vi "Read Measurement.vi"(8 "error in (no error)":errorcluster, 10 "Read From Display (0: Primary)":u16(ring) items=["Primary", "Secondary ", "Both"], 11 "VISA resource name":refnum<visa-resource-name>) -> (0 "error out":errorcluster, 1 "Secondary Display Measurement":dbl, 2 "Primary Display Measurement":dbl, 3 "VISA resource name out":refnum<visa-resource-name>, 4 "Secondary Display Units":string, 5 "Primary Display Units":string)   [LabVIEW 2015, in "Fluke 8808.lvlib"]
doc: "Reads and returns a single measurement from the instrument."
uses:
  <instrlib>/Fluke 8808/Fluke 8808.lvlib
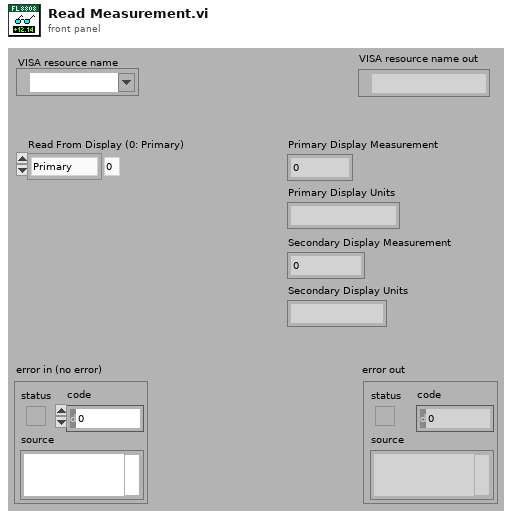
[diagram p1: front panel]
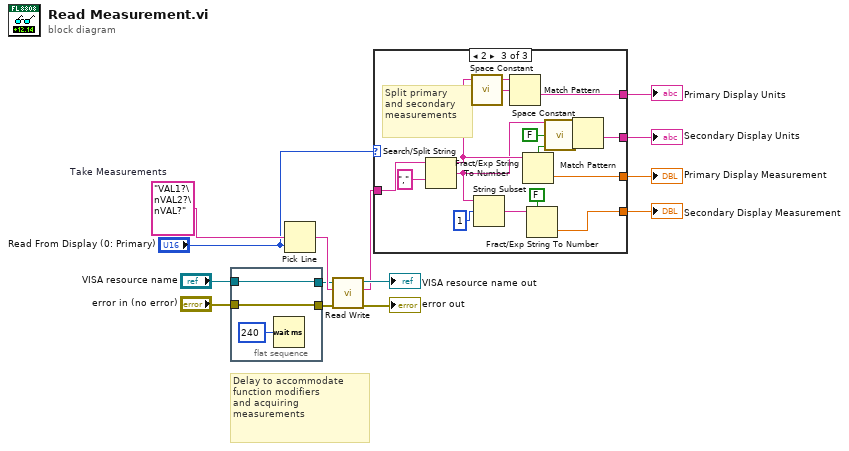
[diagram p0: block diagram]
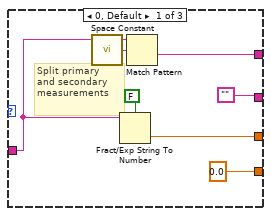
[diagram p2: hidden frame]
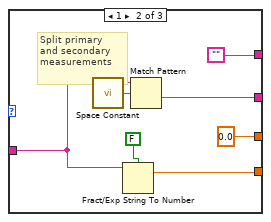
[diagram p3: hidden frame]
diagram:
  w12 = "VAL1?\nVAL2?\nVAL?"  # Take Measurements
  # "Delay to accommodate\nfunction modifiers\nand acquiring\nmeasurements"
  n1 = flat-sequence {
    tunnel: "error in (no error)" -> [w16]
    tunnel: [w16] -> w3
    tunnel: "VISA resource name" -> [w15]
    tunnel: [w15] -> w1
    frame #0 {
      n2 = Wait (ms)(milliseconds to wait=u32 240) -> ()  [unwired: 1 out]
    }
  }
  n3 = Pick Line(multi-line string=w12, line index="Read From Display (0: Primary)") -> (output string=w11:string)  [unwired: 1 in]
  n4 = call <instrlib>:"Read Write.vi"("error in (no error)"=w3, "Write String"=w11, "VISA resource name"=w1) -> ("error out"=→"error out":errorcluster, "Read Data"=w10:string, "VISA resource name out"=→"VISA resource name out":refnum<visa-resource-name>)  [unwired: 6 in]
  n5 = case shown="2" "Read From Display (0: Primary)" {
    tunnel: w10 -> [w21 w29 w45]
    tunnel: [0.0 w26 w35] -> w8
    tunnel: [w19 0.0 w36] -> w7
    tunnel: [w22 "" w41] -> w6
    tunnel: ["" w27 w37] -> w5
    frame 0, Default {
      # "Split primary\nand secondary\nmeasurements"
      n6 = call <vilib>:"Space Constant.vi"() -> ("String"=w20:string)
      n7 = Fract/Exp String To Number(use system decimal point (T)=FALSE, string=w21) -> (number=w19:dbl)  [unwired: 2 in, 1 out]
      n8 = Match Pattern(string=w21, regular expression=w20) -> (after substring=w22:string)  [unwired: 1 in, 3 out]
    }
    frame 1 {
      # "Split primary\nand secondary\nmeasurements"
      n9 = call <vilib>:"Space Constant.vi"() -> ("String"=w30:string)
      n10 = Fract/Exp String To Number(use system decimal point (T)=FALSE, string=w29) -> (number=w26:dbl)  [unwired: 2 in, 1 out]
      n11 = Match Pattern(string=w29, regular expression=w30) -> (after substring=w27:string)  [unwired: 1 in, 3 out]
    }
    frame 2 {
      # "Split primary\nand secondary\nmeasurements"
      n12 = Search/Split String(string=w45, search string/char (-)=",") -> (substring before match=w40:string, match + rest of string=w38:string)  [unwired: 1 in, 1 out]
      n13 = call <vilib>:"Space Constant.vi"() -> ("String"=w39:string)
      n14 = String Subset(string=w38, offset (0)=1) -> (substring=w42:string)  [unwired: 1 in]
      n15 = Match Pattern(string=w40, regular expression=w39) -> (after substring=w41:string)  [unwired: 1 in, 3 out]
      n16 = Fract/Exp String To Number(use system decimal point (T)=FALSE, string=w40) -> (number=w36:dbl)  [unwired: 2 in, 1 out]
      n17 = Fract/Exp String To Number(use system decimal point (T)=FALSE, string=w42) -> (number=w35:dbl)  [unwired: 2 in, 1 out]
      n18 = call <vilib>:"Space Constant.vi"() -> ("String"=w34:string)
      n19 = Match Pattern(string=w38, regular expression=w34) -> (after substring=w37:string)  [unwired: 1 in, 3 out]
    }
  }
  "Secondary Display Measurement" <- w8
  "Primary Display Measurement" <- w7
  "Primary Display Units" <- w6
  "Secondary Display Units" <- w5
